vi "fnLasViewDrawDirectRight.vi"(1 "pData":dbl[][](array[numeric])) -> (0 "返回类型":i32)   [LabVIEW 2012]
uses:
  LabView4Las.dll
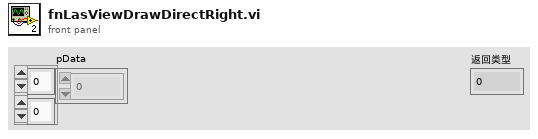
[diagram p1: front panel]
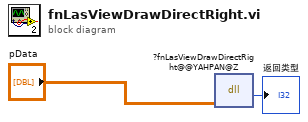
[diagram p0: block diagram]
diagram:
  n1 = dll-call lib="C:/Developer/labview/dll2/LabView4Las.dll" fn="?fnLasViewDrawDirectRight@@YAHPAN@Z"("pData"="pData") -> ("返回类型"=→"返回类型":i32)  [unwired: 4 in, 2 out]
